vi "Recieve Response with Result.vi"(4 "Finished":bool=TRUE, 6 "Result":refnum<class "Mag Lab Result.lvclass">, 8 "error in (no error)":errorcluster, 9 "Requestor":string, 10 "Requestee":string, 11 "Mag Lab Measure Controller in":refnum<class "Mag Lab Measure Controller.lvclass">) -> (0 "error out":errorcluster, 3 "Mag Lab Measure Controller out":refnum<class "Mag Lab Measure Controller.lvclass">)   [LabVIEW 2015, in "Mag Lab Measure Controller.lvclass"]
uses:
  Mag Lab Measure Controller.lvclass
  Mag Lab Result/Mag Lab Result.lvclass
  Mag Lab Root/Mag Lab Root.lvclass/Mag Lab Root.ctl
  Mag Lab Root Messages/Recieve Response with Result Msg/Recieve Response with Result Msg.lvclass/Recieve Response with Result Msg.ctl
  <vilib>/ActorFramework/Message Enqueuer/Message Enqueuer.lvclass/Message Enqueuer.ctl
  Mag Lab Measure Controller.lvclass/Mag Lab Measure Controller.ctl
  Mag Lab Measurement/Mag Lab Measurement.lvclass/Mag Lab Measurement.ctl
  <vilib>/ActorFramework/Message Enqueuer/Enqueue.vi
  <vilib>/ActorFramework/Message Priority Queue/Priority Enqueue.vi
  Mag Lab Root Messages/Recieve Response with Result Msg/Recieve Response with Result Msg.lvclass
  Compound Measurement/Compound Measurement.lvclass
  Mag Lab Measure Base/Mag Lab Measure Base.lvclass
  Mag Lab Root/Mag Lab Root.lvclass
  Mag Lab Measurement/Mag Lab Measurement.lvclass
  Mag Lab Error Handler/Mag Lab Error Handler.lvclass
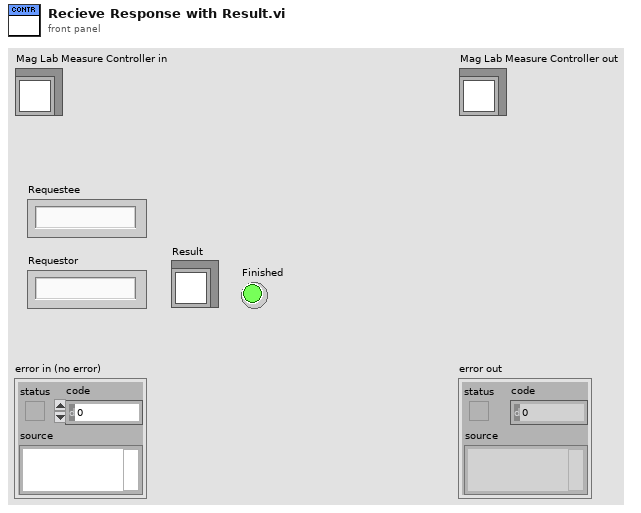
[diagram p1: front panel]
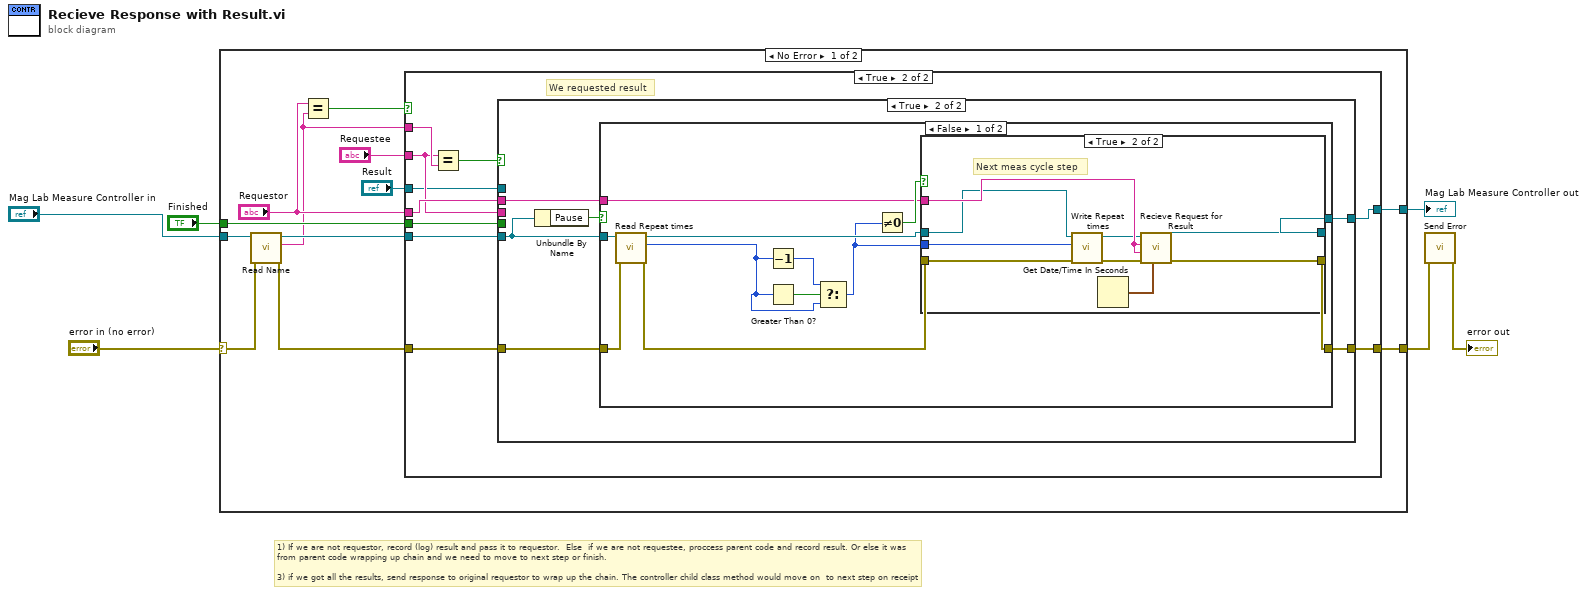
[diagram p0: block diagram]
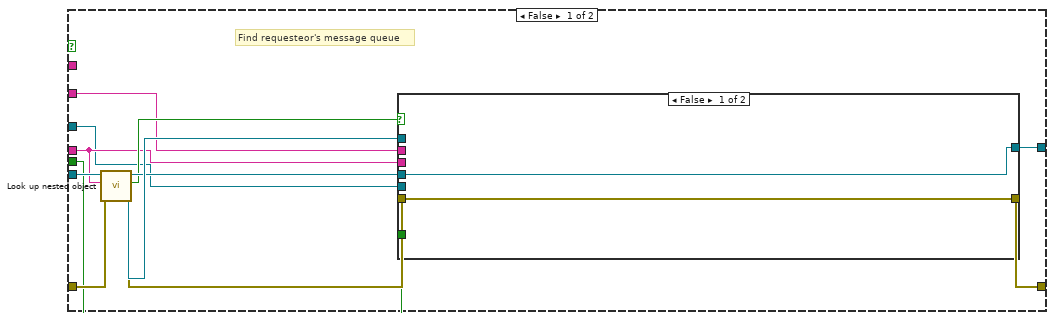
[diagram p2: hidden frame]
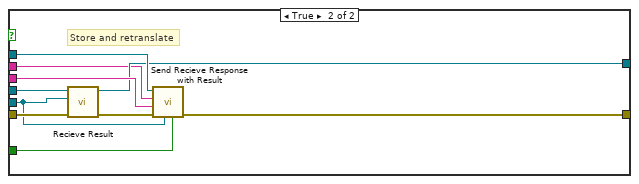
[diagram p3: hidden frame]
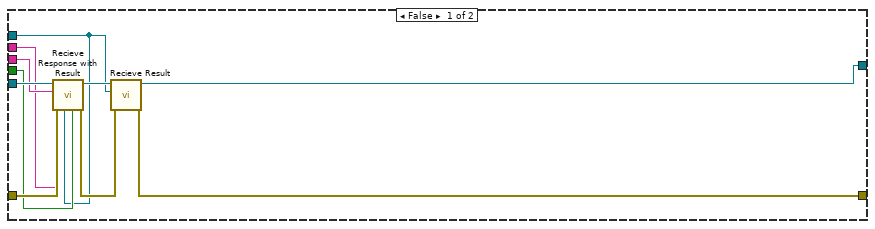
[diagram p4: hidden frame]
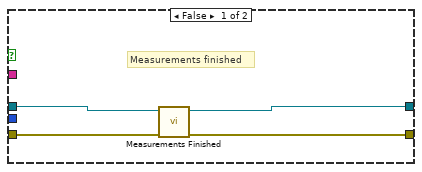
[diagram p5: hidden frame]
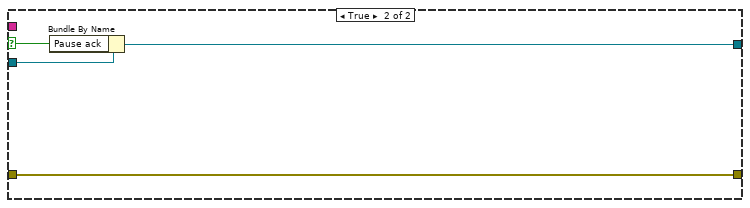
[diagram p6: hidden frame]
diagram:
  # "1) If we are not requestor, record (log) result and pass it to requestor.  Else  if we are not requestee, proccess parent code and record result. Or else it was from parent code wrapping up chain and we need to move to next step or finish.\n\n3) if we got all the results, send response to original requestor to wrap up the chain. The controller child class method would move on  to next step on receipt"
  n1 = case shown="No Error" "error in (no error)" {
    selector: "error in (no error)" -> [w14 w99]
    tunnel: [w17 w99] -> w2
    tunnel: [w18 w98] -> w4
    tunnel: "Mag Lab Measure Controller in" -> [w16 w98]
    tunnel: "Finished" -> [w11 _]
    frame No Error {
      n2 = call "Read Name.vi"("error in (no error)"=w14, "Mag Lab Root in"=w16) -> ("error out"=w13:errorcluster, "Name"=w8:string, "Mag Lab Root out"=w15:refnum<class "Mag Lab Measure Controller.lvclass">)  [unwired: 7 in]
      n3 = Equal?(x="Requestor", y=w8) -> (x = y?=w12:bool)
      n4 = case shown="True" w12 {
        tunnel: [w28 w48] -> w18
        tunnel: [w26 w49] -> w17
        tunnel: w15 -> [w24 w52]
        tunnel: "Requestor" -> [w23 w50]
        tunnel: w13 -> [w22 w51]
        tunnel: w11 -> [w21 w43]
        tunnel: "Requestee" -> [w20 w45]
        tunnel: w8 -> [_ w47]
        tunnel: "Result" -> [w19 w44]
        frame False {
          # "Find requesteor's message queue"
          n5 = call "Look up nested object.vi"("error in (no error)"=w22, "Object name"=w23, "Mag Lab Measure Base in"=w24) -> ("error out"=w27:errorcluster, "Object Queue"=w30:refnum<class "Message Enqueuer.lvclass">, "Found?"=w25:bool, "Mag Lab Measure Base out"=w29:refnum<class "Mag Lab Measure Controller.lvclass">)  [unwired: 5 in]
          n6 = case shown="False" w25 {
            tunnel: w30 -> [_ w42]
            tunnel: w23 -> [_ w41]
            tunnel: w29 -> [w32 w40]
            tunnel: [w32 w39] -> w28
            tunnel: w27 -> [w31 w38]
            tunnel: [w31 w36] -> w26
            tunnel: w21 -> [_ w35]
            tunnel: w20 -> [_ w34]
            tunnel: w19 -> [_ w33]
            frame False {
            }
            frame True {
              # "Store and retranslate"
              n7 = call-dynamic "Recieve Result.vi"("error in (no error)"=w38, "Mag Lab Result.lvclass"=w33, "Mag Lab Measure Controller in"=w40) -> ("error out"=w37:errorcluster, "Mag Lab Measure Controller out"=w39:refnum<class "Mag Lab Measure Controller.lvclass">)  [unwired: 7 in]
              n8 = call "Send Recieve Response with Result.vi"("Finished"=w35, "Result"=w33, "error in (no error)"=w37, "Requestor"=w41, "Requestee"=w34, "Message Enqueuer"=w42) -> ("error out"=w36:errorcluster)  [unwired: 4 in, 1 out]
            }
          }
        }
        frame True {
          # "We requested result"
          n9 = Equal?(x=w45, y=w47) -> (x = y?=w46:bool)
          n10 = case shown="True" w46 {
            tunnel: w52 -> [w62 w64]
            tunnel: w51 -> [w61 w68]
            tunnel: w50 -> [w59 w67]
            tunnel: [w54 w66] -> w49
            tunnel: [w55 w65] -> w48
            tunnel: w45 -> [w60 _]
            tunnel: w44 -> [w53 _]
            tunnel: w43 -> [w58 _]
            frame False {
              n11 = call-parent "Recieve Response with Result.vi"("Finished"=w58, "Result"=w53, "error in (no error)"=w61, "Requestor"=w59, "Requestee"=w60, "Compound Measurement in"=w62) -> ("error out"=w57:errorcluster, "Compound Measurement out"=w56:refnum<class "Mag Lab Measure Controller.lvclass">)  [unwired: 4 in]
              n12 = call-dynamic "Recieve Result.vi"("error in (no error)"=w57, "Mag Lab Result.lvclass"=w53, "Mag Lab Measure Controller in"=w56) -> ("error out"=w54:errorcluster, "Mag Lab Measure Controller out"=w55:refnum<class "Mag Lab Measure Controller.lvclass">)  [unwired: 7 in]
            }
            frame True {
              n13 = Unbundle By Name(w64) -> ("Pause"=w63:bool)
              n14 = case shown="False" w63 {
                selector: w63 -> [_ w97]
                tunnel: w64 -> [w80 w94]
                tunnel: w68 -> [w79 w96]
                tunnel: w67 -> [w75 _]
                tunnel: [w74 w96] -> w66
                tunnel: [w73 w95] -> w65
                frame False {
                  n15 = call "Read Repeat times.vi"("error in (no error)"=w79, "Mag Lab Measurement in"=w80) -> ("error out"=w76:errorcluster, "Repeat times"=w70:i32, "Mag Lab Measurement out"=w77:refnum<class "Mag Lab Measure Controller.lvclass">)  [unwired: 7 in]
                  n16 = Decrement(x=w70) -> (x-1=w72:i32)
                  n17 = Greater Than 0?(x=w70) -> (x > 0?=w71:bool)
                  n18 = Select(t=w72, s=w71, f=w70) -> (s? t:f=w69:i32)
                  n19 = Not Equal To 0?(x=w69) -> (x != 0?=w78:bool)
                  n20 = case shown="True" w78 {
                    tunnel: w77 -> [w84 w92]
                    tunnel: w76 -> [w82 w90]
                    tunnel: w75 -> [_ w93]
                    tunnel: w69 -> [_ w91]
                    tunnel: [w81 w88] -> w74
                    tunnel: [w83 w87] -> w73
                    frame False {
                      # "Measurements finished"
                      n21 = call-dynamic "Measurements Finished.vi"("error in (no error)"=w82, "Mag Lab Measure Controller in"=w84) -> ("error out"=w81:errorcluster, "Mag Lab Measure Controller out"=w83:refnum<class "Mag Lab Measure Controller.lvclass">)  [unwired: 8 in]
                    }
                    frame True {
                      # "Next meas cycle step"
                      n22 = call "Write Repeat times.vi"("error in (no error)"=w90, "Repeat times"=w91, "Mag Lab Measurement in"=w92) -> ("error out"=w89:errorcluster, "Mag Lab Measurement out"=w86:refnum<class "Mag Lab Measure Controller.lvclass">)  [unwired: 7 in]
                      n23 = Get Date/Time In Seconds() -> (seconds since 1Jan1904=w85:timestamp)
                      n24 = call-dynamic "Recieve Request for Result.vi"("Request time"=w85, "error in (no error)"=w89, "Requestor"=w93, "Requestee"=w93, "Mag Lab Measure Controller in"=w86) -> ("error out"=w88:errorcluster, "Mag Lab Measure Controller out"=w87:refnum<class "Mag Lab Measure Controller.lvclass">)  [unwired: 5 in]
                    }
                  }
                }
                frame True {
                  n25 = Bundle By Name(cluster=w94, "Pause ack"=w97) -> (w95:refnum<class "Mag Lab Measure Controller.lvclass">)
                }
              }
            }
          }
        }
      }
    }
    frame Error {
    }
  }
  "Mag Lab Measure Controller out" <- w4
  n26 = call "Send Error.vi"("error in (no error)"=w2) -> ("error out"=→"error out":errorcluster)  [unwired: 9 in, 1 out]
